vi "Example Callback.vi"() -> ()   [LabVIEW 2013]
uses:
  C:/tf/play/labview/Tinkerforge.dll
  Tinkerforge.dll
panel:
  out "ambient temperature (°C)":sgl format="%#_13g"
  in  "stop":bool
  out "object temperature (°C)":sgl format="%#_13g"
  in  "uid":string="kpV"
  in  "port":i32=4223
  in  "host":string="localhost"
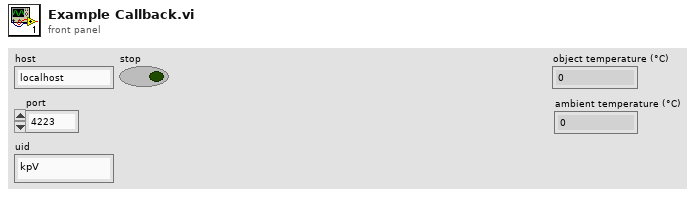
[diagram p1: front panel]
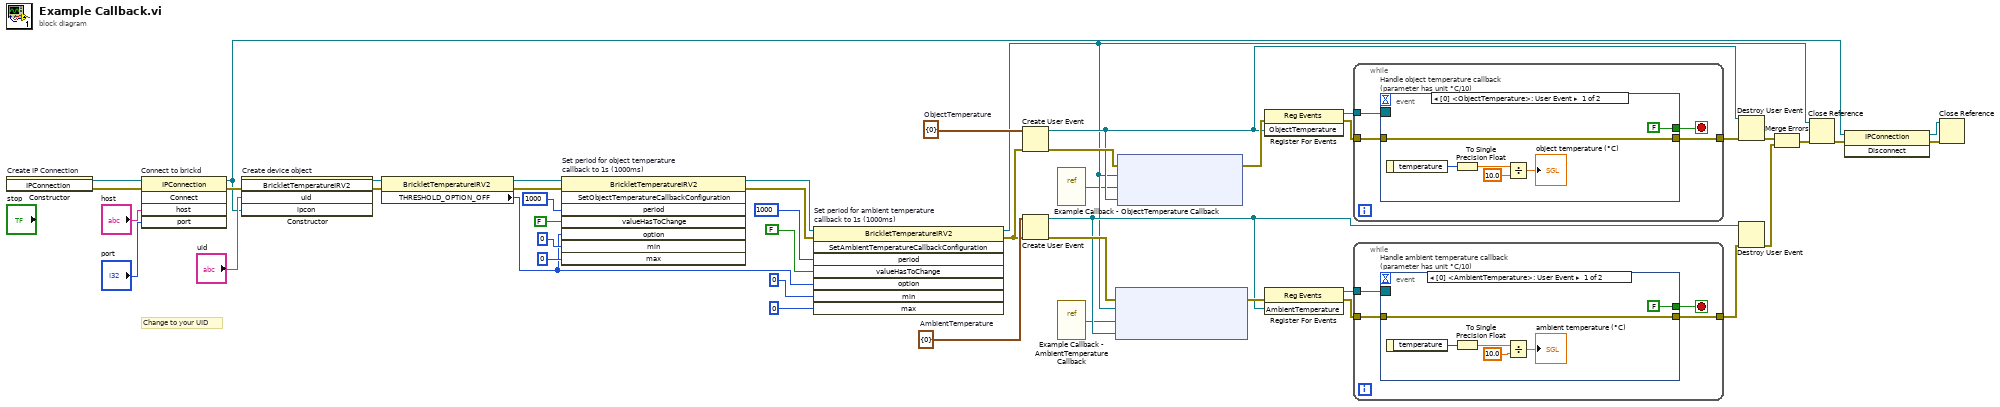
[diagram p0: block diagram]
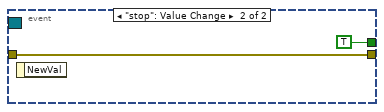
[diagram p2: hidden frame]
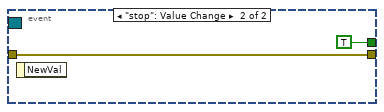
[diagram p3: hidden frame]
diagram:
  w22 = cluster{"temperature":i16} {"temperature"=0}  # AmbientTemperature
  w31 = cluster{"temperature":i16} {"temperature"=0}  # ObjectTemperature
  # "Change to your UID"
  n1 = constructor on="Create IP Connection" class="IPConnection"() -> (reference out=w46:refnum<k24>, error out=w14:errorcluster)  [unwired: 3 in, 1 out]
  n2 = invoke on="Connect to brickd" class="IPConnection" method="Connect"(reference=w46, error in=w14, "host"="host", "port"="port") -> (reference out=w39:refnum<k24>, error out=w42:errorcluster)  [unwired: 1 in, 3 out]
  n3 = constructor on="Create device object" class="BrickletTemperatureIRV2"(error in=w42, "uid"="uid", "ipcon"=w39) -> (reference out=w5:refnum<k24>, error out=w2:errorcluster)  [unwired: 2 in, 3 out]
  n4 = property class="BrickletTemperatureIRV2"(reference=w5, error in=w2) -> (reference out=w4:refnum<k24>, error out=w3:errorcluster, "THRESHOLD_OPTION_OFF"=w1:u16)
  n5 = invoke on="Set period for object temperature\ncallback to 1s (1000ms)" class="BrickletTemperatureIRV2" method="SetObjectTemperatureCallbackConfiguration"(reference=w4, error in=w3, "period"=i64 1000, "valueHasToChange"=FALSE, "option"=w1, "min"=0, "max"=0) -> (reference out=w15:refnum<k24>, error out=w16:errorcluster)  [unwired: 1 in, 6 out]
  n6 = invoke on="Set period for ambient temperature\ncallback to 1s (1000ms)" class="BrickletTemperatureIRV2" method="SetAmbientTemperatureCallbackConfiguration"(reference=w15, error in=w16, "period"=i64 1000, "valueHasToChange"=FALSE, "option"=w1, "min"=0, "max"=0) -> (reference out=w23:refnum<k24>, error out=w21:errorcluster)  [unwired: 1 in, 6 out]
  n7 = Create User Event(user event datatype=w31, error in=w21) -> (user event=w32:refnum<user-event>, error out=w37:errorcluster)
  n8 = Create User Event(user event datatype=w22, error in=w21) -> (user event=w24:refnum<user-event>, error out=w29:errorcluster)
  n9 = vi-ref "Example Callback - ObjectTemperature Callback.vi"() -> ("vi reference"=w13:refnum<vi>)
  n10 = vi-ref "Example Callback - AmbientTemperature Callback.vi"() -> ("vi reference"=w12:refnum<vi>)
  n11 = node ("Register Event Callback")(w29, w23, w12, w24) -> (w28:errorcluster)  [unwired: 1 in, 1 out]
  n12 = node ("Register Event Callback")(w37, w23, w13, w32) -> (w36:errorcluster)  [unwired: 1 in, 1 out]
  n13 = register-events(error in=w36, w32) -> (reference out=w35:refnum<event-registration>, error out=w33:errorcluster)  [unwired: 1 in]
  n14 = register-events(error in=w28, w24) -> (reference out=w27:refnum<event-registration>, error out=w25:errorcluster)  [unwired: 1 in]
  n15 = while {
    tunnel: w35 -> [w50]
    tunnel: [w49] -> w34
    tunnel: w33 -> [w48]
    stop <- w47 stop-if-true
    n16 = event "Handle object temperature callback (parameter has unit °C/10)" shown="[0] <ObjectTemperature>: User Event" {
      selector: w50 -> [_ _]
      dyn-events: _ -> [_ _]
      timeout: _ -> [_ _]
      tunnel: [w53 w57] -> w49
      tunnel: w48 -> [w53 w57]
      tunnel: [FALSE TRUE] -> w47
      event User Event {
        n17 = event-data() -> ("temperature"=w54:i16)  [unwired: 1 in]
        n18 = To Single Precision Float(number=w54) -> (single precision float=w55:sgl)
        n19 = Divide(x=w55, y=sgl 10.0) -> (x/y=→"object temperature (°C)":sgl)
      }
      event "stop": Value Change {
        n20 = event-data() -> ()  [unwired: 1 in, 1 out]
      }
    }
  }
  n21 = while {
    tunnel: w27 -> [w62]
    tunnel: [w61] -> w26
    tunnel: w25 -> [w60]
    stop <- w59 stop-if-true
    n22 = event "Handle ambient temperature callback (parameter has unit °C/10)" shown="[0] <AmbientTemperature>: User Event" {
      selector: w62 -> [_ _]
      dyn-events: _ -> [_ _]
      timeout: _ -> [_ _]
      tunnel: [w65 w69] -> w61
      tunnel: w60 -> [w65 w69]
      tunnel: [FALSE TRUE] -> w59
      event User Event {
        n23 = event-data() -> ("temperature"=w66:i16)  [unwired: 1 in]
        n24 = To Single Precision Float(number=w66) -> (single precision float=w67:sgl)
        n25 = Divide(x=w67, y=sgl 10.0) -> (x/y=→"ambient temperature (°C)":sgl)
      }
      event "stop": Value Change {
        n26 = event-data() -> ()  [unwired: 1 in, 1 out]
      }
    }
  }
  n27 = Destroy User Event(user event=w32, error in=w34) -> (error out=w19:errorcluster)
  n28 = Destroy User Event(user event=w24, error in=w26) -> (error out=w20:errorcluster)
  n29 = Merge Errors(w19, w20) -> (w18:errorcluster)
  n30 = Close Reference(reference=w23, error in (no error)=w18) -> (error out=w41:errorcluster)
  n31 = invoke class="IPConnection" method="Disconnect"(reference=w39, error in=w41) -> (reference out=w38:refnum<k24>, error out=w40:errorcluster)  [unwired: 1 in, 1 out]
  n32 = Close Reference(reference=w38, error in (no error)=w40) -> ()  [unwired: 1 out]
